vi "log.vi"(8 "error in (no error)":errorcluster, 9 "FileName":string, 10 "Path":path=path "Y:/", 11 "Data":T1 {"Power" format="%.2g"; "Voltage" format="%.2g"; "Current" format="%.2g"; "Regulator" format="%.2g"; "Extra sensor" format="%.2g"; "Cold plate" format="%.2g"; "Set point" format="%.2g"; "Main sensor" format="%.2g"}) -> (0 "error out":errorcluster, 3 "result string":string)   [LabVIEW 2013]
uses:
  controler_custer.ctl
panel:
  # "Temeprature"
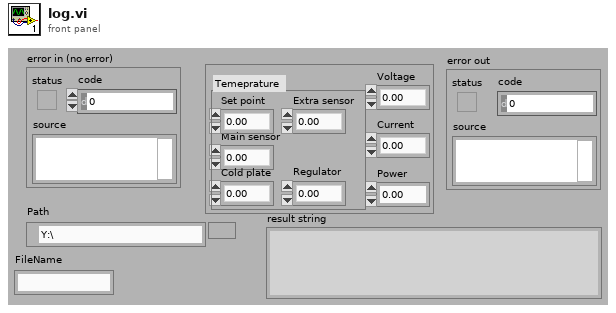
[diagram p1: front panel]
types:
  T1 = typedef "controler_custer.ctl" = cluster{"Set point":dbl, "Main sensor":dbl, "Cold plate":dbl, "Extra sensor":dbl, "Regulator":dbl, "Voltage":dbl, "Current":dbl, "Power":dbl}
  T2 = enum16{"open", "replace", "create", "open or create", "replace or create", "replace or create with confirmation"}
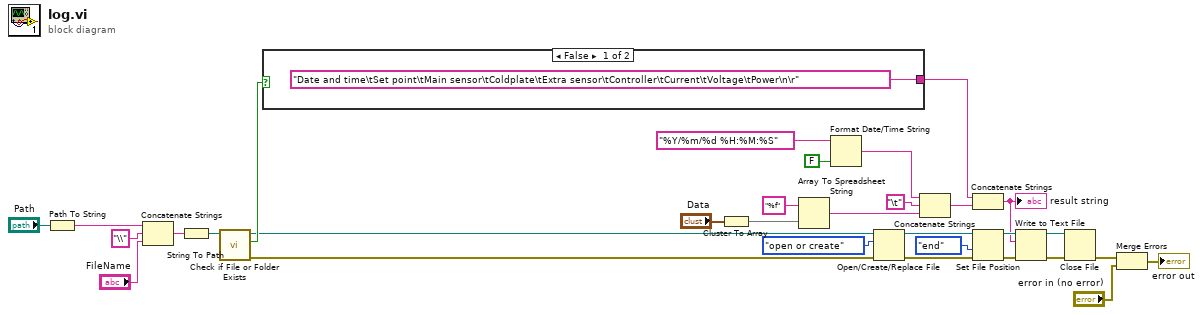
[diagram p0: block diagram]
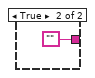
[diagram p2: hidden frame]
diagram:
  n1 = Path To String(path="Path") -> (string=w15:string)
  n2 = Concatenate Strings(w15, "\\" ("string"), "FileName") -> (w13:string)
  n3 = String To Path(string=w13) -> (path=w12:path)
  n4 = call <vilib>:"Check if File or Folder Exists.vi"("path"=w12) -> ("error out"=w4:errorcluster, "file or folder exists?"=w23:bool, "dup path"=w9:path)  [unwired: 8 in]
  n5 = case shown="False" w23 {
    tunnel: ["Date and time\tSet point\tMain sensor\tColdplate\tExtra sensor\tController\tCurrent\tVoltage\tPower\n\r" ""] -> w22
    frame False {
    }
    frame True {
    }
  }
  n6 = Cluster To Array(cluster="Data") -> (array=w18:dbl[])
  n7 = Array To Spreadsheet String(array=w18, 3:"%f" ("format string")) -> (spreadsheet string=w17:string)  [unwired: 1 in]
  n8 = Format Date/Time String(time format string (%c)="%Y/%m/%d %H:%M:%S", UTC format=FALSE ("want seconds? (F)")) -> (date/time string=w27:string)  [unwired: 1 in]
  n9 = Open/Create/Replace File(file path (use dialog)=w9, error in=w4, operation (0:open)=T2."open or create") -> (refnum out=w31:refnum<file>, error out=w8:errorcluster)  [unwired: 3 in, 1 out]
  n10 = Concatenate Strings(w27, "\t", w17) -> (w21:string)
  n11 = Concatenate Strings(w22, w21) -> (w20:string)
  "result string" <- w20
  n12 = Set File Position(refnum=w31, from (0:start)=enum16{"start", "end", "current"}."end", error in=w8) -> (refnum out=w30:refnum<file>, error out=w7:errorcluster)  [unwired: 1 in]
  n13 = Write to Text File(file (use dialog)=w30, text=w20, error in=w7) -> (refnum out=w1:refnum<file>, error out=w3:errorcluster)  [unwired: 1 in, 1 out]
  n14 = Close File(refnum=w1, error in=w3) -> (error out=w2:errorcluster)  [unwired: 1 out]
  n15 = Merge Errors(w2, "error in (no error)") -> (→"error out":errorcluster)
